vi "Trim Sensitivity - Debug.vi"(0 "TSM context":T1, 5 "Target Sensitivity (dBV)":dbl format="%#_13g", 7 "Gain":u8[](array[numeric]) format="%08b", 9 "Vbias":u8[](array[numeric]) format="%08b") -> (4 "Trimmed dB V":dbl[](array[numeric]), 15 "error out":errorcluster)   [LabVIEW 2020]
doc: "Trims sensitivity of the DUT by adjusting the Gain and Vbias values using Trim protocol"
uses:
  <vilib>/NI_TestStand_SemiconductorModule/NI_TestStand_Semiconductor_Module.lvlibp/PinMap/General/SemiconductorModuleContext.ctl
  Common/Instrument Control/Digital/TSM/TSM SSC Digital.ctl
  <vilib>/NI_TestStand_SemiconductorModule/NI_TestStand_Semiconductor_Module.lvlibp/PinMap/Digital Pattern/PinQueryContext/DigitalPatternPinQueryContext.lvclass
  Common/Instrument Control/Digital/SSC Digital/SSC Digital.ctl
  Common/Instrument Control/DCPower/TSM/TSM SSC DCPower.ctl
  <vilib>/NI_TestStand_SemiconductorModule/NI_TestStand_Semiconductor_Module.lvlibp/PinMap/PinQueryContext/MultiplePinMultipleSessionQueryContext/MultiplePinMultipleSessionQueryContext.lvclass
  Common/Instrument Control/DCPower/SSC DCPower/SSC DCPower.ctl
  Common/Instrument Control/Shared SubVIs/TSM Pin Abstraction/TSM Pin Information.ctl
  Common/Instrument Control/Shared SubVIs/TSM Pin Abstraction/TSM Pin Type Identifier.ctl
  Common/Instrument Control/Shared SubVIs/TSM Pin Abstraction/TSM Expanded Pin Information.ctl
  Common/DUT Control/Typedefs/DUT Read Commands.ctl
  Common/DUT Control/Typedefs/DUT Write Commands.ctl
  <instrlib>/niDigital/niDigital.llb/niDigital Write Static Pin State.ctl
  354e2fd9-1388-4924-804e-e9490b2eeb0b.vi
  46ecd2fd-2f0c-4e5f-b596-d218653973fe.vi
  484f7e42-a396-4691-9669-50fd76730dc7.vi
  5dce1c4a-7bee-4a31-888d-1db7ed666fe4.vi
  c53558f2-5030-41db-922a-32af9ad26e5f.vi
  354e2fd9-1388-4924-804e-e9490b2eeb0b.vi/71683651-cbc5-46e0-8522-40ce4dc1e9ef.vi
  354e2fd9-1388-4924-804e-e9490b2eeb0b.vi/5048e37d-0f89-4c33-89a7-b3c71e857334.vi
  354e2fd9-1388-4924-804e-e9490b2eeb0b.vi/0bdf4848-63d7-49b9-a33f-cfc1e4c0521b.vi
  354e2fd9-1388-4924-804e-e9490b2eeb0b.vi/b8e335d8-4854-4718-8e9f-88d363955659.vi
  Common/Instrument Control/Digital/TSM/TSM SSC Digital N Pins To M Sessions.vi
  <vilib>/NI_TestStand_SemiconductorModule/NI_TestStand_Semiconductor_Module.lvlibp/PinMap/Input Data/GetInputDataDouble.vi
  Common/Instrument Control/DCPower/SSC DCPower/Source/SSC DCPower Configure Output Enabled.vi
  Common/Instrument Control/DCPower/SSC DCPower/Source/Constant Voltage/SSC DCPower Force Voltage Array Symmetric Limits.vi
  <vilib>/NI_TestStand_SemiconductorModule/NI_TestStand_Semiconductor_Module.lvlibp/PinMap/Relay Driver/ControlRelay(s).vi
  <vilib>/NI_TestStand_SemiconductorModule/NI_TestStand_Semiconductor_Module.lvlibp/PinMap/Relay Driver/ApplyRelayConfiguration.vi
  <vilib>/Utility/High Resolution Polling Wait.vi
  <vilib>/NI_TestStand_SemiconductorModule/NI_TestStand_Semiconductor_Module.lvlibp/PinMap/General/Publish/PublishDataDoubleFunctionalTest.vi
  Common/Instrument Control/Digital/SSC Digital/Static/SSC Digital Write Static.vi
  <vilib>/NI_TestStand_SemiconductorModule/NI_TestStand_Semiconductor_Module.lvlibp
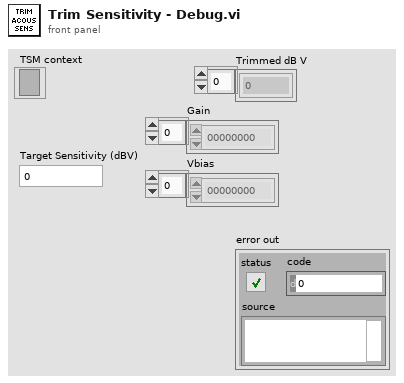
[diagram p1: front panel]
types:
  T1 = typedef "NI_TestStand_Semiconductor_Module.lvlibp/SemiconductorModuleContext.ctl" = refnum<k7>
  T2 = typedef "TSM SSC Digital.ctl" = cluster{"Pin Query Context":refnum<class "DigitalPatternPinQueryContext.lvclass">, "SSC":T3[], "Site Numbers":i32[], "Pins":tag[]}
  T3 = typedef "SSC Digital.ctl" = cluster{"Session":refnum<k15>, "Channel List":string, "Site List":string}
  T4 = typedef "TSM SSC DCPower.ctl" = cluster{"Pin Query Context":refnum<class "MultiplePinMultipleSessionQueryContext.lvclass">, "SSC":T5[], "Site Numbers":i32[], "Pins":T6[], "Pins Expanded":T8[]}
  T5 = typedef "SSC DCPower.ctl" = cluster{"Session":refnum<k15>, "Chan":string, "Channel List":string}
  T6 = typedef "TSM Pin Information.ctl" = cluster{"Pin":tag, "Type":T7, "Count":i32}
  T7 = typedef "TSM Pin Type Identifier.ctl" = enum8{"DUT Pin", "System Pin", "Pin Group", "Not Determined"}
  T8 = typedef "TSM Expanded Pin Information.ctl" = cluster{"Pin":tag, "Type":T7, "Index":i32}
  T9 = cluster{"OTP Pins":T2, "SMU_VDD_MERGED":T4, "PreTrim Sensitivity":dbl[], "PreTrimOTP":u8[]}
  T10 = typedef "DUT Read Commands.ctl" = enum16{"Read Reg and Timeout", "Read OTP and Timeout"}
  T11 = typedef "DUT Write Commands.ctl" = enum16{"Write Reg and Timeout", "Write Reg and Nmode Cmd", "Program OTP"}
  T12 = typedef "niDigital Write Static Pin State.ctl" = u8
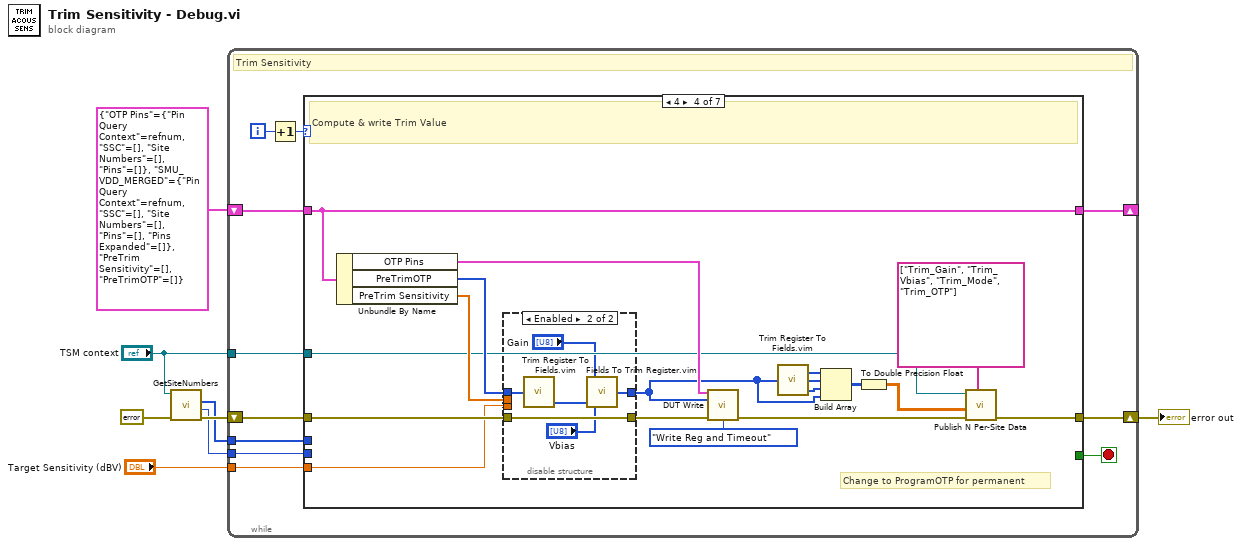
[diagram p0: block diagram]
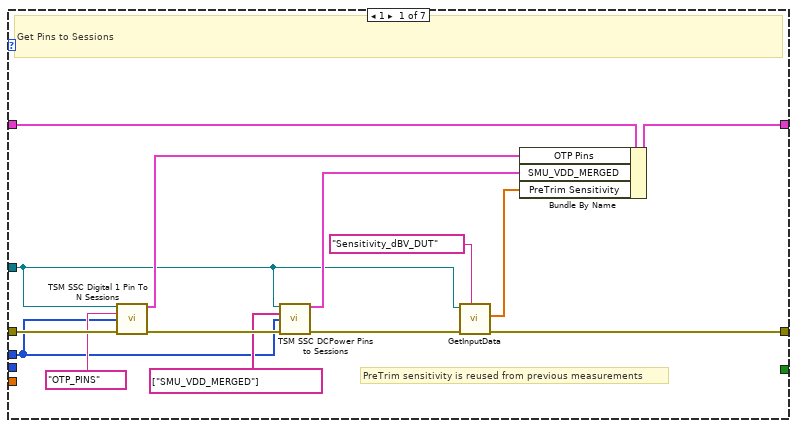
[diagram p2: hidden frame]
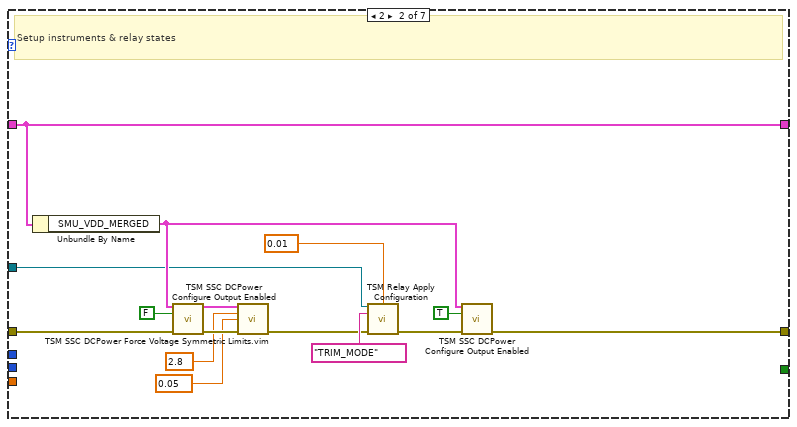
[diagram p3: hidden frame]
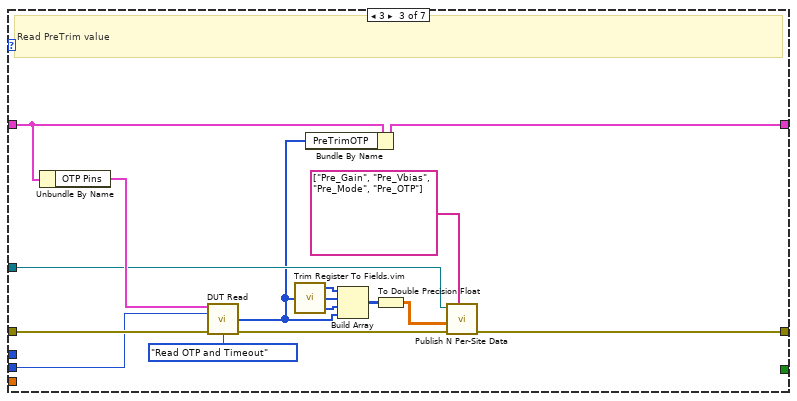
[diagram p4: hidden frame]
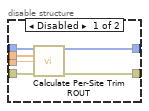
[diagram p5: hidden frame]
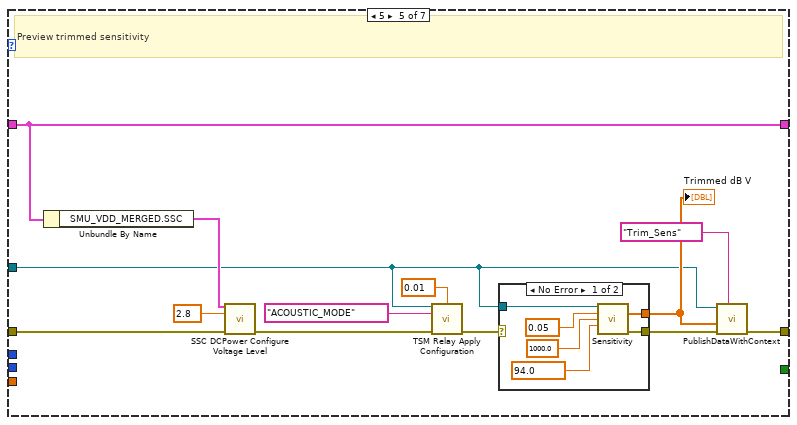
[diagram p6: hidden frame]
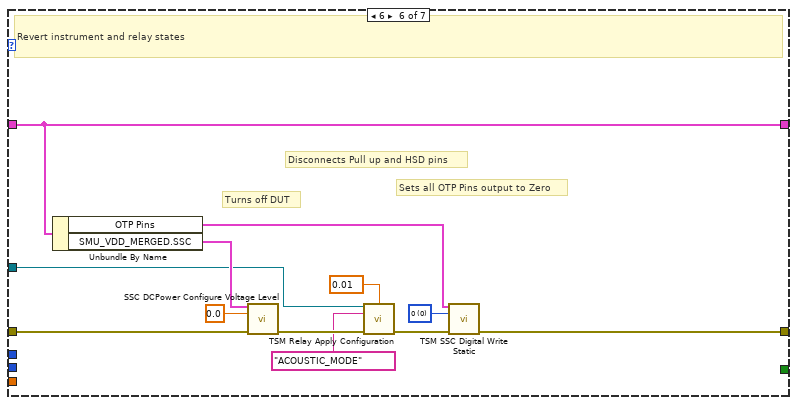
[diagram p8: hidden frame]
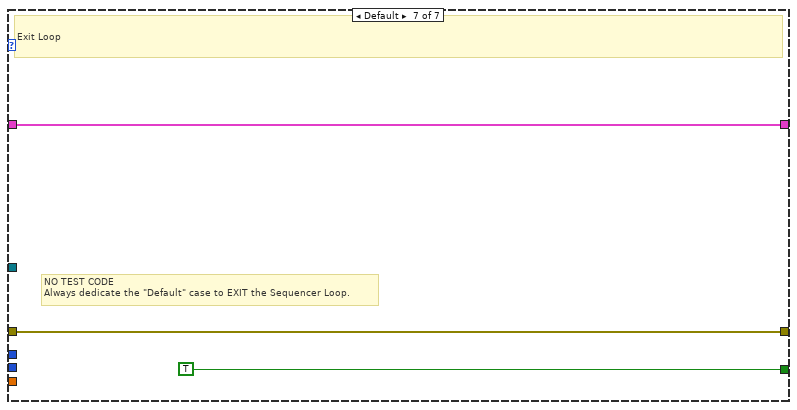
[diagram p9: hidden frame]
diagram:
  n1 = call <vilib>:"GetSiteNumbers.vi"("error in (no error)"=errorcluster {"status"=FALSE, "code"=0, "source"=""} ("error in"), "Semiconductor Module Context"="TSM context") -> ("error out"=w5:errorcluster, "Number Of Sites"=w1:i32, "Site Numbers"=w3:i32[])  [unwired: 6 in, 1 out]
  n2 = while {
    shift-right: [w17] -> w8
    shift-left: w5 -> [w18]
    tunnel: "TSM context" -> [w15]
    shift-right: [w12] -> _
    shift-left: T9 {"OTP Pins"={"Pin Query Context"=refnum, "SSC"=[], "Site Numbers"=[], "Pins"=[]}, "SMU_VDD_MERGED"={"Pin Query Context"=refnum, "SSC"=[], "Site Numbers"=[], "Pins"=[], "Pins Expanded"=[]}, "PreTrim Sensitivity"=[], "PreTrimOTP"=[]} -> [w13]
    tunnel: w3 -> [w11]
    tunnel: "Target Sensitivity (dBV)" -> [w10]
    tunnel: w1 -> [w9]
    i -> [w19]
    stop <- w14 stop-if-true
    # "Trim Sensitivity"
    n3 = Increment(x=w19) -> (x+1=w16:i32)
    n4 = case shown="4" w16 {
      tunnel: [w24 w46 w49 w66 w98 w115 w128] -> w17
      tunnel: w18 -> [w33 w48 w63 w82 w105 w126 w128]
      tunnel: w15 -> [w22 w35 w53 w67 w96 w120 _]
      tunnel: [_ _ _ _ _ _ TRUE] -> w14
      tunnel: w13 -> [w32 w44 w61 w79 w101 w123 w127]
      tunnel: [w29 w44 w51 w79 w101 w123 w127] -> w12
      tunnel: w11 -> [w21 _ _ _ _ _ _]
      tunnel: w10 -> [_ _ _ w80 _ _ _]
      tunnel: w9 -> [_ _ w62 _ _ _ _]
      frame 1 {
        # "PreTrim sensitivity is reused from previous measurements"
        # "Get Pins to Sessions"
        n5 = call "TSM SSC Digital 1 Pin To N Sessions.vi"("TSM context"=w22, "Pin"=tag "OTP_PINS", "Site Numbers"=w21, "error in"=w33) -> ("Digital TSM Out"=w28:T2, "error out"=w31:errorcluster)  [unwired: 10 in]
        n6 = call "TSM SSC DCPower Pins to Sessions.vi"("TSM context"=w22, "Pins"=tag[] ["SMU_VDD_MERGED"], "Site Numbers"=w21, "error in"=w31) -> ("DCPower TSM Out"=w26:T4, "error out"=w23:errorcluster)  [unwired: 10 in]
        n7 = call-poly <vilib>:"GetInputData.vi"("Input Data Id"=tag "Sensitivity_dBV_DUT", "error in (no error)"=w23, "Semiconductor Module Context"=w22) -> ("error out"=w24:errorcluster, "Data Out"=w20:dbl[])  [unwired: 6 in, 1 out]
        n8 = Bundle By Name(cluster=w32, "OTP Pins"=w28, "SMU_VDD_MERGED"=w26, "PreTrim Sensitivity"=w20) -> (w29:T9)
      }
      frame 2 {
        # "Setup instruments & relay states"
        n9 = Unbundle By Name(w44) -> ("SMU_VDD_MERGED"=w39:T4)
        n10 = call "TSM SSC DCPower Configure Output Enabled.vi"("DCPower TSM in"=w39, "Output Enabled"=FALSE, "error in"=w48) -> ("DCPower TSM out"=w43:T4, "error out"=w47:errorcluster)  [unwired: 11 in]
        n11 = call "TSM SSC DCPower Force Voltage Symmetric Limits.vim"("DCPower TSM in"=w43, "Voltage Level (V)"=2.8, "Current Limit (A)"=0.05, "error in"=w47) -> ("error out"=w36:errorcluster)  [unwired: 10 in, 1 out]
        n12 = call "TSM Relay Apply Configuration.vi"("TSM Context"=w35, "Settling Time (0s)"=0.01, "Relay Configuration"=tag "TRIM_MODE", "error in (no error)"=w36) -> ("error out"=w38:errorcluster)  [unwired: 11 in]
        n13 = call "TSM SSC DCPower Configure Output Enabled.vi"("DCPower TSM in"=w39, "Output Enabled"=TRUE, "error in"=w38) -> ("error out"=w46:errorcluster)  [unwired: 11 in, 1 out]
      }
      frame 3 {
        # "Read PreTrim value"
        n14 = Unbundle By Name(w61) -> ("OTP Pins"=w60:T2)
        n15 = call "DUT Read.vi"("Digital TSM In"=w60, "Number Of Sites"=w62, "error in (no error)"=w63, "Operation"=DUT_Read_Commands."Read OTP and Timeout") -> ("Per Site Read Data"=w50:u8[], "error out"=w54:errorcluster)  [unwired: 8 in, 2 out]
        n16 = call "Trim Register To Fields.vim"("ROUT"=w50) -> ("Mode"=w57:u8[], "Vbias"=w58:u8[], "Gain"=w59:u8[])  [unwired: 2 in]
        n17 = Bundle By Name(cluster=w61, "PreTrimOTP"=w50) -> (w51:T9)
        n18 = Build Array(w59, w58, w57, w50) -> (w56:u8[][])
        n19 = To Double Precision Float(number=w56) -> (double precision float=w52:dbl[][])
        n20 = call "Publish N Per-Site Data.vi"("Published Data Id"=tag[] ["Pre_Gain", "Pre_Vbias", "Pre_Mode", "Pre_OTP"], "error in (no error)"=w54, "Data In"=w52, "Semiconductor Module Context"=w53) -> ("error out"=w49:errorcluster)  [unwired: 6 in, 1 out]
      }
      frame 4 {
        # "Change to ProgramOTP for permanent"
        # "Compute & write Trim Value"
        n21 = Unbundle By Name(w79) -> ("OTP Pins"=w76:T2, "PreTrimOTP"=w78:u8[], "PreTrim Sensitivity"=w77:dbl[])
        n22 = disable-structure shown="Enabled" {
          disable-tunnel: w82 -> [w88 w93]
          disable-tunnel: [w87 w93] -> w81
          disable-tunnel: w80 -> [w86 _]
          disable-tunnel: w78 -> [w85 w92]
          disable-tunnel: w77 -> [w84 _]
          disable-tunnel: [w83 w94] -> w68
          frame Disabled {
            n23 = call "Calculate Per-Site Trim ROUT.vi"("Per Site ROUT In"=w85, "Per-Site Cur Sensitivity(dBV)"=w84, "Target Sensitivity(dBV)"=w86, "error in (no error)"=w88) -> ("Per Site ROUT Out"=w83:u8[], "error out"=w87:errorcluster)  [unwired: 10 in]
          }
          frame Enabled {
            n24 = call "Trim Register To Fields.vim"("ROUT"=w92) -> ("Mode"=w91:u8[])  [unwired: 2 in, 2 out]
            n25 = call "Fields To Trim Register.vim"("Mode"=w91, "Vbias"="Vbias", "Gain"="Gain") -> ("ROUT"=w94:u8[])  [unwired: 2 in]
          }
        }
        n26 = call "DUT Write.vi"("Digital TSM In"=w76, "Per Site Data In"=w68, "error in (no error)"=w81, "Operation"=DUT_Write_Commands."Write Reg and Timeout") -> ("error out"=w70:errorcluster)  [unwired: 8 in, 3 out]
        n27 = call "Trim Register To Fields.vim"("ROUT"=w68) -> ("Mode"=w73:u8[], "Vbias"=w74:u8[], "Gain"=w75:u8[])  [unwired: 2 in]
        n28 = Build Array(w75, w74, w73, w68) -> (w72:u8[][])
        n29 = To Double Precision Float(number=w72) -> (double precision float=w69:dbl[][])
        n30 = call "Publish N Per-Site Data.vi"("Published Data Id"=tag[] ["Trim_Gain", "Trim_Vbias", "Trim_Mode", "Trim_OTP"], "error in (no error)"=w70, "Data In"=w69, "Semiconductor Module Context"=w67) -> ("error out"=w66:errorcluster)  [unwired: 6 in, 1 out]
      }
      frame 5 {
        # "Preview trimmed sensitivity"
        n31 = Unbundle By Name(w101) -> ("SMU_VDD_MERGED.SSC"=w100:T5[])
        n32 = call "SSC DCPower Configure Voltage Level.vi"("DCPower SSC in"=w100, "Voltage Level (V)"=2.8, "error in"=w105) -> ("error out"=w102:errorcluster)  [unwired: 11 in, 1 out]
        n33 = call "TSM Relay Apply Configuration.vi"("TSM Context"=w96, "Settling Time (0s)"=0.01, "Relay Configuration"=tag "ACOUSTIC_MODE", "error in (no error)"=w102) -> ("error out"=w104:errorcluster)  [unwired: 11 in]
        n34 = case shown="No Error" w104 {
          selector: w104 -> [_ w114]
          tunnel: [w113 w114] -> w103
          tunnel: [w112 _] -> w97
          tunnel: w96 -> [w108 _]
          frame No Error {
            n35 = call "Sensitivity.vi"("TSM context"=w108, "Capture Duration (s)"=0.05, "Frequency"=1000.0, "dB SPL"=94.0) -> ("dB V"=w112:dbl[], "error out"=w113:errorcluster)  [unwired: 9 in, 1 out]
          }
          frame Error {
          }
        }
        "Trimmed dB V" <- w97
        n36 = call-poly <vilib>:"PublishDataWithContext.vi"("Published Data Id"=tag "Trim_Sens", "error in (no error)"=w103, "Data In"=w97, "Semiconductor Module Context"=w96) -> ("error out"=w98:errorcluster)  [unwired: 6 in, 1 out]
      }
      frame 6 {
        w118 = T12 0 items=["0"=0, "1"=1, "X"=5] ("State")
        # "Sets all OTP Pins output to Zero"
        # "Disconnects Pull up and HSD pins"
        # "Turns off DUT"
        # "Revert instrument and relay states"
        n37 = Unbundle By Name(w123) -> ("OTP Pins"=w117:T2, "SMU_VDD_MERGED.SSC"=w122:T5[])
        n38 = call "SSC DCPower Configure Voltage Level.vi"("DCPower SSC in"=w122, "Voltage Level (V)"=0.0, "error in"=w126) -> ("error out"=w125:errorcluster)  [unwired: 11 in, 1 out]
        n39 = call "TSM Relay Apply Configuration.vi"("TSM Context"=w120, "Settling Time (0s)"=0.01, "Relay Configuration"=tag "ACOUSTIC_MODE", "error in (no error)"=w125) -> ("error out"=w116:errorcluster)  [unwired: 11 in]
        n40 = call "TSM SSC Digital Write Static.vi"("Digital TSM in"=w117, "State"=w118, "error in"=w116) -> ("error out"=w115:errorcluster)  [unwired: 11 in, 1 out]
      }
      frame Default {
        # "NO TEST CODE\nAlways dedicate the \"Default\" case to EXIT the Sequencer Loop."
        # "Exit Loop"
      }
    }
  }
  "error out" <- w8
